vi "Save.vi"(8 "error in (no error)":errorcluster, 10 "Text":string, 11 "Experiment2D in":refnum<class "Experiment2D.lvclass">) -> (0 "error out":errorcluster, 3 "Experiment2D out":refnum<class "Experiment2D.lvclass">)   [LabVIEW 2014, in "Experiment2D.lvclass"]
uses:
  Experiment2D.lvclass
  Data/Data2D/Data2D.lvclass
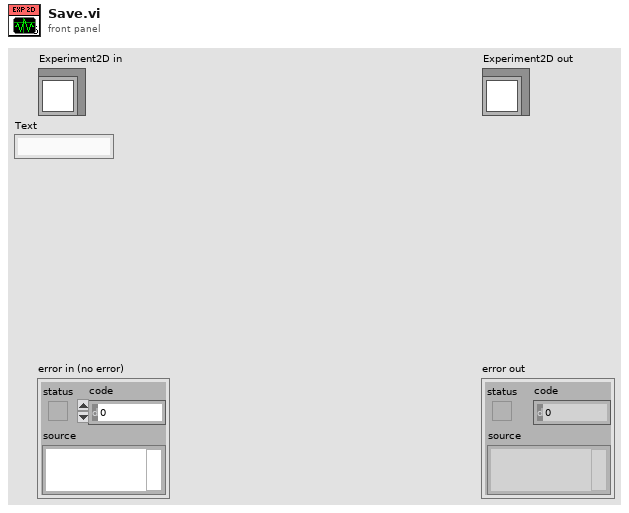
[diagram p1: front panel]
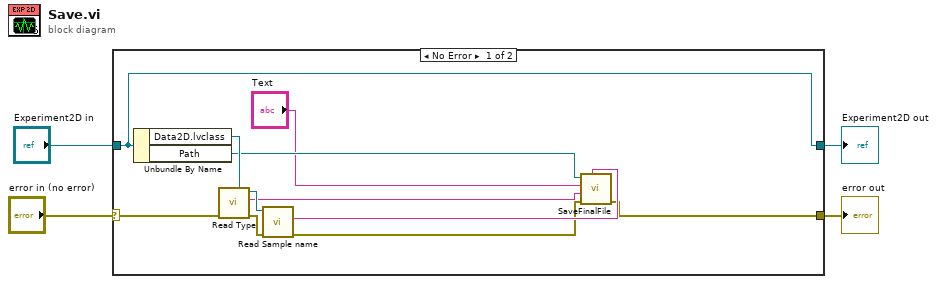
[diagram p0: block diagram]
diagram:
  n1 = case shown="No Error" "error in (no error)" {
    selector: "error in (no error)" -> [w12 w17]
    tunnel: [w11 w16] -> w2
    tunnel: "Experiment2D in" -> [w11 w16]
    tunnel: [w5 w17] -> w1
    frame No Error {
      n2 = Unbundle By Name(w11) -> ("Data2D.lvclass"=w13:refnum<class "Data2D.lvclass">, "Path"=w10:path)
      n3 = call-dynamic "Read Type.vi"("error in (no error)"=w12, "Data2D in"=w13) -> ("error out"=w14:errorcluster, "Type"=w8:string, "Data2D out"=w15:refnum<class "Data2D.lvclass">)  [unwired: 7 in]
      n4 = call-dynamic "Read Sample name.vi"("error in (no error)"=w14, "Data2D in"=w15) -> ("error out"=w6:errorcluster, "Sample name"=w7:string)  [unwired: 7 in, 1 out]
      n5 = call "SaveFinalFile.vi"("Sample name"=w7, "error in (no error)"=w6, "Type"=w8, "Text"="Text", "Path"=w10) -> ("error out"=w5:errorcluster)  [unwired: 6 in]
    }
    frame Error {
    }
  }
  "error out" <- w1
  "Experiment2D out" <- w2
